vi "GetProperties.vi"(8 "error in":errorcluster, 11 "GraphScale in":refnum<class "GraphScale.lvclass">) -> (0 "error out":errorcluster, 3 "GraphScale out":refnum<class "GraphScale.lvclass">)   [LabVIEW 2014, in "GraphScale.lvclass"]
uses:
  GraphScale.lvclass
  GraphScale.lvclass/GraphScale.ctl
  Scale/Scale.lvclass
  Text/Text.lvclass
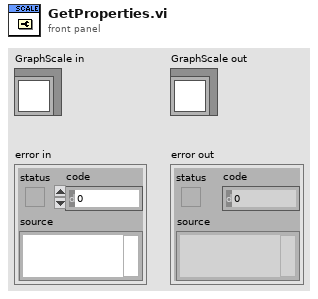
[diagram p1: front panel]
types:
  T1 = typedef "LVOffsetAndMultiplierTypeDef.ctl" = cluster{"Offset":dbl, "Multiplier":dbl}
  T2 = typedef "LVMajorAndMinorColorsTypeDef.ctl" = cluster{"Major Color":u32, "Minor Color":u32}
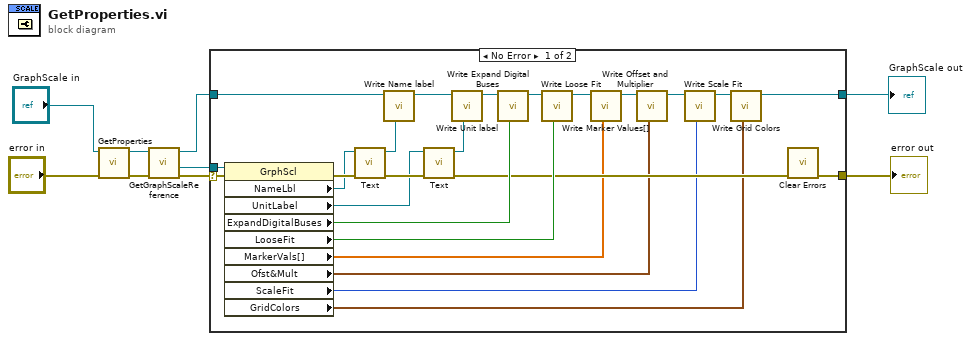
[diagram p0: block diagram]
diagram:
  n1 = call-parent "GetProperties.vi"("error in"="error in", "Scale in"="GraphScale in") -> ("error out"=w6:errorcluster, "Scale out"=w7:refnum<class "GraphScale.lvclass">)  [unwired: 8 in]
  n2 = call "GetGraphScaleReference.vi"("error in"=w6, "GraphScale in"=w7) -> ("error out"=w5:errorcluster, "graph scale reference"=w3:refnum<vi>, "GraphScale out"=w4:refnum<class "GraphScale.lvclass">)  [unwired: 7 in]
  n3 = case shown="No Error" w5 {
    selector: w5 -> [w33 w35]
    tunnel: w4 -> [w25 w36]
    tunnel: w3 -> [w34 _]
    tunnel: [w15 w35] -> w1
    tunnel: [w14 w36] -> w2
    frame No Error {
      n4 = property class="GrphScl"(reference=w34, error in=w33) -> (error out=w32:errorcluster, "NameLbl"=w31:refnum<vi>, "UnitLabel"=w29:refnum<vi>, "ExpandDigitalBuses"=w23:bool, "LooseFit"=w21:bool, "MarkerVals[]"=w10:dbl[], "Ofst&Mult"=w11:T1, "ScaleFit"=w12:u8, "GridColors"=w13:T2)  [unwired: 1 out]
      n5 = call "Text.vi"("error in"=w32, "Gen Refnum"=w31) -> ("error out"=w30:errorcluster, "Text out"=w27:refnum<class "Text.lvclass">)  [unwired: 8 in]
      n6 = call "Write Name label.vi"("Name label"=w27, "GraphScale in"=w25) -> ("GraphScale out"=w26:refnum<class "GraphScale.lvclass">)  [unwired: 7 in]
      n7 = call "Text.vi"("error in"=w30, "Gen Refnum"=w29) -> ("error out"=w16:errorcluster, "Text out"=w28:refnum<class "Text.lvclass">)  [unwired: 8 in]
      n8 = call "Write Unit label.vi"("Unit label"=w28, "GraphScale in"=w26) -> ("GraphScale out"=w24:refnum<class "GraphScale.lvclass">)  [unwired: 7 in]
      n9 = call "Write Expand Digital Buses.vi"("Expand Digital Buses"=w23, "GraphScale in"=w24) -> ("GraphScale out"=w22:refnum<class "GraphScale.lvclass">)  [unwired: 7 in]
      n10 = call "Write Loose Fit.vi"("Loose Fit"=w21, "GraphScale in"=w22) -> ("GraphScale out"=w20:refnum<class "GraphScale.lvclass">)  [unwired: 7 in]
      n11 = call "Write Marker Values[].vi"("Marker Values[]"=w10, "GraphScale in"=w20) -> ("GraphScale out"=w19:refnum<class "GraphScale.lvclass">)  [unwired: 7 in]
      n12 = call "Write Offset and Multiplier.vi"("Offset and Multiplier"=w11, "GraphScale in"=w19) -> ("GraphScale out"=w18:refnum<class "GraphScale.lvclass">)  [unwired: 7 in]
      n13 = call "Write Scale Fit.vi"("Scale Fit"=w12, "GraphScale in"=w18) -> ("GraphScale out"=w17:refnum<class "GraphScale.lvclass">)  [unwired: 7 in]
      n14 = call "Write Grid Colors.vi"("Grid Colors"=w13, "GraphScale in"=w17) -> ("GraphScale out"=w14:refnum<class "GraphScale.lvclass">)  [unwired: 7 in]
      n15 = call <vilib>:"Clear Errors.vi"("error in (no error)"=w16) -> ("error out"=w15:errorcluster)  [unwired: 5 in, 1 out]
    }
    frame Error {
    }
  }
  "error out" <- w1
  "GraphScale out" <- w2
